vi "BMU诊断标定.vi"(8 "CAN端口":u16(ring), 9 "设备索引号":u16(ring), 10 "CAN卡类型":u32(ring)=21) -> ()   [LabVIEW 2013] (continued)
          event "保存主板参数": Value Change {
            n1903 = event-data() -> ("NewVal"=w2321:bool)  [unwired: 6 out]
            n1904 = case shown="真" w2321 {
              tunnel: w2325 -> [w2327 w2332]
              tunnel: [w2327 w2331] -> w2324
              tunnel: w2323 -> [w2326 w2330]
              tunnel: [w2326 w2329] -> w2322
              frame False {
              }
              frame True {
                n1905 = call <vilib>:"Set Busy.vi"() -> ()  [unwired: 4 in, 8 out]
                n1906 = Enqueue Element(queue=w2332, element="写配置文件", error in (no error)=w2330) -> (queue out=w2331:refnum<queue>, error out=w2329:errorcluster)  [unwired: 2 out]
              }
            }
          }
          event "继电器全开": Value Change {
            n1907 = event-data() -> ("NewVal"=w2333:bool)  [unwired: 6 out]
            n1908 = case shown="真" w2333 {
              tunnel: w2333 -> [_ w2336]
              frame False {
              }
              frame True {
                n1909 = stacked-sequence {
                  tunnel: w2336 -> [_ w2346 _]
                  frame #0 {
                    w2337 = FALSE ("清BUFF")
                    n1910 = local write "正级继电器"(w2337) -> ()
                    n1911 = local write "负级继电器"(w2337) -> ()
                    n1912 = local write "充电继电器"(w2337) -> ()
                    n1913 = local write "加热继电器"(w2337) -> ()
                    n1914 = local write "风机继电器"(w2337) -> ()
                    n1915 = local write "预充电继电器"(w2337) -> ()
                    n1916 = local write "继电器超时处理"(FALSE ("继电器超时处理")) -> ()
                    n1917 = local write "主从选择"(enum32{"主板", "从板"}."主板" ("主从选择")) -> ()
                    n1918 = local write "清BUFF"(FALSE ("清BUFF")) -> ()
                  }
                  frame #1 {
                    n1919 = case shown="真" w2346 {
                      selector: w2346 -> [_ w2361]
                      frame False {
                      }
                      frame True {
                        w2357 = 256.0 ("y")
                        w2348 = u32 1 ("命令序号")
                        w2347 = u8 192 ("命令")
                        n1920 = local read "动作保持时间"() -> (w2358:dbl)
                        n1921 = Quotient & Remainder(x=w2358, y=w2357) -> (x-y*floor(x/y)=w2350:dbl, floor(x/y)=w2354:dbl)
                        n1922 = Quotient & Remainder(x=w2354, y=w2357) -> (x-y*floor(x/y)=w2351:dbl, floor(x/y)=w2355:dbl)
                        n1923 = Quotient & Remainder(x=w2355, y=w2357) -> (x-y*floor(x/y)=w2352:dbl, floor(x/y)=w2356:dbl)
                        n1924 = local read "设备索引号"() -> (w2365:u16)
                        n1925 = local read "CAN卡类型"() -> (w2366:u32)
                        n1926 = local read "CAN端口"() -> (w2364:u16)
                        n1927 = Boolean To (0,1)(Boolean=w2361) -> (0, 1=w2359:i16)
                        n1928 = Quotient & Remainder(x=w2356, y=w2357) -> (x-y*floor(x/y)=w2353:dbl)  [unwired: 1 out]
                        n1929 = Build Array(i16 170 ("元素"), w2359, w2353, w2352, w2351, w2350, 0.0 ("元素")) -> (w2362:dbl[])
                        n1930 = call "多帧发送机制(EV05).vi"("can卡类型"=w2366, "设备索引号"=w2365, "CAN端口"=w2364, "命令"=w2347, "板号"=u8 0, "命令序号"=w2348, "输入数据"=w2362) -> ()  [unwired: 1 in, 12 out]
                        n1931 = local write "命令序号"(w2348) -> ()
                        n1932 = local write "命令"(w2347) -> ()
                      }
                    }
                    n1933 = local write "控制1"(TRUE ("控制1")) -> ()
                    n1934 = local write "写?"(FALSE ("写?")) -> ()
                    n1935 = local write "消除"(TRUE ("消除")) -> ()
                    n1936 = global write "EV05全局变量1.vi" "流控帧 2"(TRUE ("流控帧 2")) -> ()
                    n1937 = global write "EV05全局变量1.vi" "流控帧"(FALSE ("流控帧")) -> ()
                  }
                  frame #2 {
                    n1938 = flat-sequence {
                      tunnel: [w2368] -> w2367
                      tunnel: w2367 -> [w2375]
                      frame #0 {
                        n1939 = while {
                          tunnel: [w2369] -> w2368
                          i -> [w2373]
                          stop <- w2370 stop-if-true
                          n1940 = local read "继电器超时处理"() -> (w2369:bool)
                          n1941 = Greater Or Equal?(x=w2373, y=20) -> (x >= y?=w2371:bool)
                          n1942 = Wait Until Next ms Multiple(millisecond multiple=u32 100 ("毫秒倍数")) -> ()  [unwired: 1 out]
                          n1943 = Or(x=w2369, y=w2371) -> (x .or. y?=w2370:bool)
                        }
                      }
                      frame #1 {
                        n1944 = case shown="真" w2375 {
                          frame False {
                            n1945 = One Button Dialog(message="继电器处理超时" ("消息"), button name ("OK")="是" ("按钮名称（“确定”）")) -> ()  [unwired: 1 out]
                          }
                          frame True {
                            w2378 = TRUE ("清BUFF")
                            n1946 = local write "正级继电器"(w2378) -> ()
                            n1947 = local write "负级继电器"(w2378) -> ()
                            n1948 = local write "充电继电器"(w2378) -> ()
                            n1949 = local write "加热继电器"(w2378) -> ()
                            n1950 = local write "风机继电器"(w2378) -> ()
                            n1951 = local write "预充电继电器"(w2378) -> ()
                          }
                        }
                      }
                    }
                  }
                }
              }
            }
          }
          event "继电器全关": Value Change {
            n1952 = event-data() -> ("NewVal"=w2379:bool)  [unwired: 6 out]
            n1953 = case shown="真" w2379 {
              tunnel: w2379 -> [_ w2382]
              frame False {
              }
              frame True {
                n1954 = stacked-sequence {
                  tunnel: w2382 -> [_ w2392 _]
                  frame #0 {
                    w2383 = TRUE ("清BUFF")
                    n1955 = local write "正级继电器"(w2383) -> ()
                    n1956 = local write "负级继电器"(w2383) -> ()
                    n1957 = local write "充电继电器"(w2383) -> ()
                    n1958 = local write "加热继电器"(w2383) -> ()
                    n1959 = local write "风机继电器"(w2383) -> ()
                    n1960 = local write "预充电继电器"(w2383) -> ()
                    n1961 = local write "继电器超时处理"(FALSE ("继电器超时处理")) -> ()
                    n1962 = local write "主从选择"(enum32{"主板", "从板"}."主板" ("主从选择")) -> ()
                    n1963 = global write "EV05全局变量1.vi" "流控帧"(FALSE ("流控帧")) -> ()
                    n1964 = local write "清BUFF"(FALSE ("清BUFF")) -> ()
                  }
                  frame #1 {
                    n1965 = case shown="真" w2392 {
                      selector: w2392 -> [_ w2407]
                      frame False {
                      }
                      frame True {
                        w2403 = 256.0 ("y")
                        w2394 = u32 1 ("命令序号")
                        w2393 = u8 192 ("命令")
                        n1966 = local read "动作保持时间"() -> (w2404:dbl)
                        n1967 = Quotient & Remainder(x=w2404, y=w2403) -> (x-y*floor(x/y)=w2396:dbl, floor(x/y)=w2400:dbl)
                        n1968 = Quotient & Remainder(x=w2400, y=w2403) -> (x-y*floor(x/y)=w2397:dbl, floor(x/y)=w2401:dbl)
                        n1969 = Quotient & Remainder(x=w2401, y=w2403) -> (x-y*floor(x/y)=w2398:dbl, floor(x/y)=w2402:dbl)
                        n1970 = local read "设备索引号"() -> (w2411:u16)
                        n1971 = local read "CAN卡类型"() -> (w2412:u32)
                        n1972 = local read "CAN端口"() -> (w2410:u16)
                        n1973 = Boolean To (0,1)(Boolean=w2407) -> (0, 1=w2405:i16)
                        n1974 = Quotient & Remainder(x=w2402, y=w2403) -> (x-y*floor(x/y)=w2399:dbl)  [unwired: 1 out]
                        n1975 = Build Array(i16 85 ("元素"), w2405, w2399, w2398, w2397, w2396, 0.0 ("元素")) -> (w2408:dbl[])
                        n1976 = call "多帧发送机制(EV05).vi"("can卡类型"=w2412, "设备索引号"=w2411, "CAN端口"=w2410, "命令"=w2393, "板号"=u8 0, "命令序号"=w2394, "输入数据"=w2408) -> ()  [unwired: 1 in, 12 out]
                        n1977 = local write "命令序号"(w2394) -> ()
                        n1978 = local write "命令"(w2393) -> ()
                      }
                    }
                    n1979 = local write "控制1"(TRUE ("控制1")) -> ()
                    n1980 = local write "写?"(FALSE ("写?")) -> ()
                    n1981 = local write "消除"(TRUE ("消除")) -> ()
                    n1982 = global write "EV05全局变量1.vi" "流控帧 2"(TRUE ("流控帧 2")) -> ()
                  }
                  frame #2 {
                    n1983 = flat-sequence {
                      tunnel: [w2414] -> w2413
                      tunnel: w2413 -> [w2421]
                      frame #0 {
                        n1984 = while {
                          tunnel: [w2415] -> w2414
                          i -> [w2419]
                          stop <- w2416 stop-if-true
                          n1985 = local read "继电器超时处理"() -> (w2415:bool)
                          n1986 = Greater Or Equal?(x=w2419, y=20) -> (x >= y?=w2417:bool)
                          n1987 = Wait Until Next ms Multiple(millisecond multiple=u32 100 ("毫秒倍数")) -> ()  [unwired: 1 out]
                          n1988 = Or(x=w2415, y=w2417) -> (x .or. y?=w2416:bool)
                        }
                      }
                      frame #1 {
                        n1989 = case shown="真" w2421 {
                          frame False {
                            n1990 = One Button Dialog(message="继电器处理超时" ("消息"), button name ("OK")="是" ("按钮名称（“确定”）")) -> ()  [unwired: 1 out]
                          }
                          frame True {
                            w2424 = FALSE ("清BUFF")
                            n1991 = local write "正级继电器"(w2424) -> ()
                            n1992 = local write "负级继电器"(w2424) -> ()
                            n1993 = local write "充电继电器"(w2424) -> ()
                            n1994 = local write "加热继电器"(w2424) -> ()
                            n1995 = local write "风机继电器"(w2424) -> ()
                            n1996 = local write "预充电继电器"(w2424) -> ()
                          }
                        }
                      }
                    }
                  }
                }
              }
            }
          }
          event "控制按键全为开": Value Change {
            n1997 = event-data() -> ("NewVal"=w2425:bool)  [unwired: 6 out]
            n1998 = case shown="真" w2425 {
              frame False {
              }
              frame True {
                w2426 = TRUE ("正级继电器")
                n1999 = local write "加热继电器(从)"(w2426) -> ()
                n2000 = local write "风机继电器(从)"(w2426) -> ()
                n2001 = local write "DO1 2"(w2426) -> ()
                n2002 = local write "DO1"(w2426) -> ()
                n2003 = local write "DO2"(w2426) -> ()
                n2004 = local write "正级继电器"(w2426) -> ()
                n2005 = local write "负级继电器"(w2426) -> ()
                n2006 = local write "加热继电器"(w2426) -> ()
                n2007 = local write "预充电继电器"(w2426) -> ()
                n2008 = local write "充电继电器"(w2426) -> ()
                n2009 = local write "风机继电器"(w2426) -> ()
              }
            }
          }
          event "控制按键全为关": Value Change {
            n2010 = event-data() -> ("NewVal"=w2427:bool)  [unwired: 6 out]
            n2011 = case shown="真" w2427 {
              frame False {
              }
              frame True {
                w2428 = FALSE ("正级继电器")
                n2012 = local write "加热继电器(从)"(w2428) -> ()
                n2013 = local write "风机继电器(从)"(w2428) -> ()
                n2014 = local write "DO1 2"(w2428) -> ()
                n2015 = local write "DO1"(w2428) -> ()
                n2016 = local write "DO2"(w2428) -> ()
                n2017 = local write "正级继电器"(w2428) -> ()
                n2018 = local write "负级继电器"(w2428) -> ()
                n2019 = local write "加热继电器"(w2428) -> ()
                n2020 = local write "预充电继电器"(w2428) -> ()
                n2021 = local write "充电继电器"(w2428) -> ()
                n2022 = local write "风机继电器"(w2428) -> ()
              }
            }
          }
          event "正级继电器": Value Change {
            n2023 = event-data() -> ("NewVal"=w2429:bool)  [unwired: 6 out]
            n2024 = stacked-sequence {
              tunnel: w2429 -> [_ w2442 _]
              frame #0 {
                w2432 = FALSE ("清BUFF")
                n2025 = local write "继电器超时处理"(FALSE ("继电器超时处理")) -> ()
                n2026 = local write "主从选择"(enum32{"主板", "从板"}."主板" ("主从选择")) -> ()
                n2027 = local write "正级继电器 12"(w2432) -> ()
                n2028 = local write "清BUFF"(w2432) -> ()
              }
              frame #1 {
                n2029 = case shown="假" w2442 {
                  selector: w2442 -> [w2457 w2477]
                  tunnel: [w2456 w2476] -> w2441
                  tunnel: [w2444 w2464] -> w2436
                  frame False {
                    w2452 = 256.0 ("y")
                    w2444 = u32 1 ("命令序号")
                    w2456 = u8 192 ("命令")
                    n2030 = local read "动作保持时间"() -> (w2453:dbl)
                    n2031 = Quotient & Remainder(x=w2453, y=w2452) -> (x-y*floor(x/y)=w2445:dbl, floor(x/y)=w2449:dbl)
                    n2032 = Quotient & Remainder(x=w2449, y=w2452) -> (x-y*floor(x/y)=w2446:dbl, floor(x/y)=w2450:dbl)
                    n2033 = Quotient & Remainder(x=w2450, y=w2452) -> (x-y*floor(x/y)=w2447:dbl, floor(x/y)=w2451:dbl)
                    n2034 = local read "设备索引号"() -> (w2461:u16)
                    n2035 = local read "CAN卡类型"() -> (w2462:u32)
                    n2036 = local read "CAN端口"() -> (w2460:u16)
                    n2037 = Boolean To (0,1)(Boolean=w2457) -> (0, 1=w2454:i16)
                    n2038 = Quotient & Remainder(x=w2451, y=w2452) -> (x-y*floor(x/y)=w2448:dbl)  [unwired: 1 out]
                    n2039 = Build Array(i16 1 ("元素"), w2454, w2448, w2447, w2446, w2445, 0.0 ("元素")) -> (w2458:dbl[])
                    n2040 = call "多帧发送机制(EV05).vi"("can卡类型"=w2462, "设备索引号"=w2461, "CAN端口"=w2460, "命令"=w2456, "板号"=u8 0, "命令序号"=w2444, "输入数据"=w2458) -> ()  [unwired: 1 in, 12 out]
                  }
                  frame True {
                    w2472 = 256.0 ("y")
                    w2464 = u32 1 ("命令序号")
                    w2476 = u8 192 ("命令")
                    n2041 = local read "动作保持时间"() -> (w2473:dbl)
                    n2042 = Quotient & Remainder(x=w2473, y=w2472) -> (x-y*floor(x/y)=w2465:dbl, floor(x/y)=w2469:dbl)
                    n2043 = Quotient & Remainder(x=w2469, y=w2472) -> (x-y*floor(x/y)=w2466:dbl, floor(x/y)=w2470:dbl)
                    n2044 = Quotient & Remainder(x=w2470, y=w2472) -> (x-y*floor(x/y)=w2467:dbl, floor(x/y)=w2471:dbl)
                    n2045 = local read "设备索引号"() -> (w2481:u16)
                    n2046 = local read "CAN卡类型"() -> (w2482:u32)
                    n2047 = local read "CAN端口"() -> (w2480:u16)
                    n2048 = Boolean To (0,1)(Boolean=w2477) -> (0, 1=w2474:i16)
                    n2049 = Quotient & Remainder(x=w2471, y=w2472) -> (x-y*floor(x/y)=w2468:dbl)  [unwired: 1 out]
                    n2050 = Build Array(i16 1 ("元素"), w2474, w2468, w2467, w2466, w2465, 0.0 ("元素")) -> (w2478:dbl[])
                    n2051 = call "多帧发送机制(EV05).vi"("can卡类型"=w2482, "设备索引号"=w2481, "CAN端口"=w2480, "命令"=w2476, "板号"=u8 0, "命令序号"=w2464, "输入数据"=w2478) -> ()  [unwired: 1 in, 12 out]
                  }
                }
                n2052 = local write "命令序号"(w2436) -> ()
                n2053 = local write "命令"(w2441) -> ()
                n2054 = local write "控制1"(TRUE ("控制1")) -> ()
                n2055 = local write "写?"(FALSE ("写?")) -> ()
                n2056 = global write "EV05全局变量1.vi" "流控帧"(FALSE ("流控帧")) -> ()
                n2057 = local write "消除"(TRUE ("消除")) -> ()
                n2058 = global write "EV05全局变量1.vi" "流控帧 2"(TRUE ("流控帧 2")) -> ()
              }
              frame #2 {
                n2059 = flat-sequence {
                  tunnel: [w2484] -> w2483
                  tunnel: w2483 -> [w2491]
                  frame #0 {
                    n2060 = while {
                      tunnel: [w2485] -> w2484
                      i -> [w2489]
                      stop <- w2486 stop-if-true
                      n2061 = local read "继电器超时处理"() -> (w2485:bool)
                      n2062 = Greater Or Equal?(x=w2489, y=20) -> (x >= y?=w2487:bool)
                      n2063 = Wait Until Next ms Multiple(millisecond multiple=u32 100 ("毫秒倍数")) -> ()  [unwired: 1 out]
                      n2064 = Or(x=w2485, y=w2487) -> (x .or. y?=w2486:bool)
                    }
                  }
                  frame #1 {
                    n2065 = case shown="假" w2491 {
                      frame False {
                        n2066 = local read "正级继电器"() -> (w2493:bool)
                        n2067 = Not(x=w2493) -> (.not. x?=w2492:bool)
                        n2068 = local write "正级继电器"(w2492) -> ()
                        n2069 = One Button Dialog(message="继电器处理超时" ("消息"), button name ("OK")="是" ("按钮名称（“确定”）")) -> ()  [unwired: 1 out]
                      }
                      frame True {
                      }
                    }
                  }
                }
              }
            }
          }
          event "负级继电器": Value Change {
            n2070 = event-data() -> ("NewVal"=w2496:bool)  [unwired: 6 out]
            n2071 = stacked-sequence {
              tunnel: w2496 -> [_ w2509 _]
              frame #0 {
                w2499 = FALSE ("继电器超时处理")
                n2072 = local write "继电器超时处理"(w2499) -> ()
                n2073 = local write "正级继电器 2"(w2499) -> ()
                n2074 = local write "主从选择"(enum32{"主板", "从板"}."主板" ("主从选择")) -> ()
              }
              frame #1 {
                n2075 = case shown="假" w2509 {
                  selector: w2509 -> [w2523 w2543]
                  tunnel: [w2522 w2542] -> w2508
                  tunnel: [w2511 w2531] -> w2503
                  frame False {
                    w2519 = 256.0 ("y")
                    w2511 = u32 1 ("命令序号")
                    w2522 = u8 192 ("命令")
                    n2076 = local read "动作保持时间"() -> (w2520:dbl)
                    n2077 = Quotient & Remainder(x=w2520, y=w2519) -> (x-y*floor(x/y)=w2512:dbl, floor(x/y)=w2516:dbl)
                    n2078 = Quotient & Remainder(x=w2516, y=w2519) -> (x-y*floor(x/y)=w2513:dbl, floor(x/y)=w2517:dbl)
                    n2079 = Quotient & Remainder(x=w2517, y=w2519) -> (x-y*floor(x/y)=w2514:dbl, floor(x/y)=w2518:dbl)
                    n2080 = Quotient & Remainder(x=w2518, y=w2519) -> (x-y*floor(x/y)=w2515:dbl)  [unwired: 1 out]
                    n2081 = Boolean To (0,1)(Boolean=w2523) -> (0, 1=w2521:i16)
                    n2082 = local read "设备索引号"() -> (w2528:u16)
                    n2083 = local read "CAN卡类型"() -> (w2529:u32)
                    n2084 = local read "CAN端口"() -> (w2527:u16)
                    n2085 = Build Array(i16 2 ("元素"), w2521, w2515, w2514, w2513, w2512, 0.0 ("元素")) -> (w2525:dbl[])
                    n2086 = call "多帧发送机制(EV05).vi"("can卡类型"=w2529, "设备索引号"=w2528, "CAN端口"=w2527, "命令"=w2522, "板号"=u8 0, "命令序号"=w2511, "输入数据"=w2525) -> ()  [unwired: 1 in, 12 out]
                  }
                  frame True {
                    w2539 = 256.0 ("y")
                    w2531 = u32 1 ("命令序号")
                    w2542 = u8 192 ("命令")
                    n2087 = local read "动作保持时间"() -> (w2540:dbl)
                    n2088 = Quotient & Remainder(x=w2540, y=w2539) -> (x-y*floor(x/y)=w2532:dbl, floor(x/y)=w2536:dbl)
                    n2089 = Quotient & Remainder(x=w2536, y=w2539) -> (x-y*floor(x/y)=w2533:dbl, floor(x/y)=w2537:dbl)
                    n2090 = Quotient & Remainder(x=w2537, y=w2539) -> (x-y*floor(x/y)=w2534:dbl, floor(x/y)=w2538:dbl)
                    n2091 = Quotient & Remainder(x=w2538, y=w2539) -> (x-y*floor(x/y)=w2535:dbl)  [unwired: 1 out]
                    n2092 = Boolean To (0,1)(Boolean=w2543) -> (0, 1=w2541:i16)
                    n2093 = local read "设备索引号"() -> (w2548:u16)
                    n2094 = local read "CAN卡类型"() -> (w2549:u32)
                    n2095 = local read "CAN端口"() -> (w2547:u16)
                    n2096 = Build Array(i16 2 ("元素"), w2541, w2535, w2534, w2533, w2532, 0.0 ("元素")) -> (w2545:dbl[])
                    n2097 = call "多帧发送机制(EV05).vi"("can卡类型"=w2549, "设备索引号"=w2548, "CAN端口"=w2547, "命令"=w2542, "板号"=u8 0, "命令序号"=w2531, "输入数据"=w2545) -> ()  [unwired: 1 in, 12 out]
                  }
                }
                n2098 = local write "命令"(w2508) -> ()
                n2099 = local write "命令序号"(w2503) -> ()
                n2100 = local write "清BUFF"(FALSE ("清BUFF")) -> ()
                n2101 = global write "EV05全局变量1.vi" "流控帧"(FALSE ("流控帧")) -> ()
                n2102 = local write "控制1"(TRUE ("控制1")) -> ()
                n2103 = global write "EV05全局变量1.vi" "流控帧 2"(TRUE ("流控帧 2")) -> ()
                n2104 = local write "写?"(FALSE ("写?")) -> ()
                n2105 = local write "消除"(TRUE ("消除")) -> ()
              }
              frame #2 {
                n2106 = flat-sequence {
                  tunnel: [w2551] -> w2550
                  tunnel: w2550 -> [w2558]
                  frame #0 {
                    n2107 = while {
                      tunnel: [w2552] -> w2551
                      i -> [w2556]
                      stop <- w2553 stop-if-true
                      n2108 = local read "继电器超时处理"() -> (w2552:bool)
                      n2109 = Greater Or Equal?(x=w2556, y=20) -> (x >= y?=w2554:bool)
                      n2110 = Wait Until Next ms Multiple(millisecond multiple=u32 100 ("毫秒倍数")) -> ()  [unwired: 1 out]
                      n2111 = Or(x=w2552, y=w2554) -> (x .or. y?=w2553:bool)
                    }
                  }
                  frame #1 {
                    n2112 = case shown="假" w2558 {
                      frame False {
                        n2113 = local read "负级继电器"() -> (w2559:bool)
                        n2114 = Not(x=w2559) -> (.not. x?=w2560:bool)
                        n2115 = local write "负级继电器"(w2560) -> ()
                        n2116 = One Button Dialog(message="继电器处理超时" ("消息"), button name ("OK")="是" ("按钮名称（“确定”）")) -> ()  [unwired: 1 out]
                      }
                      frame True {
                      }
                    }
                  }
                }
              }
            }
          }
          event "预充电继电器": Value Change {
            n2117 = event-data() -> ("NewVal"=w2563:bool)  [unwired: 6 out]
            n2118 = stacked-sequence {
              tunnel: w2563 -> [_ w2576 _]
              frame #0 {
                w2567 = FALSE ("继电器超时处理")
                n2119 = local write "继电器超时处理"(w2567) -> ()
                n2120 = local write "正级继电器 3"(w2567) -> ()
                n2121 = global write "EV05全局变量1.vi" "流控帧"(FALSE ("流控帧")) -> ()
                n2122 = local write "主从选择"(enum32{"主板", "从板"}."主板" ("主从选择")) -> ()
              }
              frame #1 {
                n2123 = case shown="假" w2576 {
                  selector: w2576 -> [w2590 w2610]
                  tunnel: [w2589 w2609] -> w2575
                  tunnel: [w2578 w2598] -> w2570
                  frame False {
                    w2586 = 256.0 ("y")
                    w2578 = u32 1 ("命令序号")
                    w2589 = u8 192 ("命令")
                    n2124 = local read "动作保持时间"() -> (w2587:dbl)
                    n2125 = Quotient & Remainder(x=w2587, y=w2586) -> (x-y*floor(x/y)=w2579:dbl, floor(x/y)=w2583:dbl)
                    n2126 = Quotient & Remainder(x=w2583, y=w2586) -> (x-y*floor(x/y)=w2580:dbl, floor(x/y)=w2584:dbl)
                    n2127 = Quotient & Remainder(x=w2584, y=w2586) -> (x-y*floor(x/y)=w2581:dbl, floor(x/y)=w2585:dbl)
                    n2128 = Quotient & Remainder(x=w2585, y=w2586) -> (x-y*floor(x/y)=w2582:dbl)  [unwired: 1 out]
                    n2129 = Boolean To (0,1)(Boolean=w2590) -> (0, 1=w2588:i16)
                    n2130 = local read "设备索引号"() -> (w2595:u16)
                    n2131 = local read "CAN卡类型"() -> (w2596:u32)
                    n2132 = local read "CAN端口"() -> (w2594:u16)
                    n2133 = Build Array(i16 3 ("元素"), w2588, w2582, w2581, w2580, w2579, 0.0 ("元素")) -> (w2592:dbl[])
                    n2134 = call "多帧发送机制(EV05).vi"("can卡类型"=w2596, "设备索引号"=w2595, "CAN端口"=w2594, "命令"=w2589, "板号"=u8 0, "命令序号"=w2578, "输入数据"=w2592) -> ()  [unwired: 1 in, 12 out]
                  }
                  frame True {
                    w2606 = 256.0 ("y")
                    w2598 = u32 1 ("命令序号")
                    w2609 = u8 192 ("命令")
                    n2135 = local read "动作保持时间"() -> (w2607:dbl)
                    n2136 = Quotient & Remainder(x=w2607, y=w2606) -> (x-y*floor(x/y)=w2599:dbl, floor(x/y)=w2603:dbl)
                    n2137 = Quotient & Remainder(x=w2603, y=w2606) -> (x-y*floor(x/y)=w2600:dbl, floor(x/y)=w2604:dbl)
                    n2138 = Quotient & Remainder(x=w2604, y=w2606) -> (x-y*floor(x/y)=w2601:dbl, floor(x/y)=w2605:dbl)
                    n2139 = Quotient & Remainder(x=w2605, y=w2606) -> (x-y*floor(x/y)=w2602:dbl)  [unwired: 1 out]
                    n2140 = Boolean To (0,1)(Boolean=w2610) -> (0, 1=w2608:i16)
                    n2141 = local read "设备索引号"() -> (w2615:u16)
                    n2142 = local read "CAN卡类型"() -> (w2616:u32)
                    n2143 = local read "CAN端口"() -> (w2614:u16)
                    n2144 = Build Array(i16 3 ("元素"), w2608, w2602, w2601, w2600, w2599, 0.0 ("元素")) -> (w2612:dbl[])
                    n2145 = call "多帧发送机制(EV05).vi"("can卡类型"=w2616, "设备索引号"=w2615, "CAN端口"=w2614, "命令"=w2609, "板号"=u8 0, "命令序号"=w2598, "输入数据"=w2612) -> ()  [unwired: 1 in, 12 out]
                  }
                }
                n2146 = local write "命令序号"(w2570) -> ()
                n2147 = local write "清BUFF"(FALSE ("清BUFF")) -> ()
                n2148 = local write "控制1"(TRUE ("控制1")) -> ()
                n2149 = global write "EV05全局变量1.vi" "流控帧 2"(TRUE ("流控帧 2")) -> ()
                n2150 = local write "消除"(TRUE ("消除")) -> ()
                n2151 = local write "命令"(w2575) -> ()
                n2152 = local write "写?"(FALSE ("写?")) -> ()
              }
              frame #2 {
                n2153 = flat-sequence {
                  tunnel: [w2618] -> w2617
                  tunnel: w2617 -> [w2625]
                  frame #0 {
                    n2154 = while {
                      tunnel: [w2619] -> w2618
                      i -> [w2623]
                      stop <- w2620 stop-if-true
                      n2155 = local read "继电器超时处理"() -> (w2619:bool)
                      n2156 = Greater Or Equal?(x=w2623, y=20) -> (x >= y?=w2621:bool)
                      n2157 = Wait Until Next ms Multiple(millisecond multiple=u32 100 ("毫秒倍数")) -> ()  [unwired: 1 out]
                      n2158 = Or(x=w2619, y=w2621) -> (x .or. y?=w2620:bool)
                    }
                  }
                  frame #1 {
                    n2159 = case shown="假" w2625 {
                      frame False {
                        n2160 = local read "预充电继电器"() -> (w2626:bool)
                        n2161 = Not(x=w2626) -> (.not. x?=w2627:bool)
                        n2162 = local write "预充电继电器"(w2627) -> ()
                        n2163 = One Button Dialog(message="继电器处理超时" ("消息"), button name ("OK")="是" ("按钮名称（“确定”）")) -> ()  [unwired: 1 out]
                      }
                      frame True {
                      }
                    }
                  }
                }
              }
            }
          }
          event "加热继电器": Value Change {
            n2164 = event-data() -> ("NewVal"=w2630:bool)  [unwired: 6 out]
            n2165 = stacked-sequence {
              tunnel: w2630 -> [_ w2643 _]
              frame #0 {
                w2634 = FALSE ("继电器超时处理")
                n2166 = local write "继电器超时处理"(w2634) -> ()
                n2167 = local write "正级继电器 5"(w2634) -> ()
                n2168 = global write "EV05全局变量1.vi" "流控帧"(FALSE ("流控帧")) -> ()
                n2169 = local write "主从选择"(enum32{"主板", "从板"}."主板" ("主从选择")) -> ()
              }
              frame #1 {
                n2170 = case shown="假" w2643 {
                  selector: w2643 -> [w2657 w2677]
                  tunnel: [w2656 w2676] -> w2642
                  tunnel: [w2645 w2665] -> w2637
                  frame False {
                    w2653 = 256.0 ("y")
                    w2645 = u32 1 ("命令序号")
                    w2656 = u8 192 ("命令")
                    n2171 = local read "动作保持时间"() -> (w2654:dbl)
                    n2172 = Quotient & Remainder(x=w2654, y=w2653) -> (x-y*floor(x/y)=w2646:dbl, floor(x/y)=w2650:dbl)
                    n2173 = Quotient & Remainder(x=w2650, y=w2653) -> (x-y*floor(x/y)=w2647:dbl, floor(x/y)=w2651:dbl)
                    n2174 = Quotient & Remainder(x=w2651, y=w2653) -> (x-y*floor(x/y)=w2648:dbl, floor(x/y)=w2652:dbl)
                    n2175 = Quotient & Remainder(x=w2652, y=w2653) -> (x-y*floor(x/y)=w2649:dbl)  [unwired: 1 out]
                    n2176 = Boolean To (0,1)(Boolean=w2657) -> (0, 1=w2655:i16)
                    n2177 = local read "设备索引号"() -> (w2662:u16)
                    n2178 = local read "CAN卡类型"() -> (w2663:u32)
                    n2179 = local read "CAN端口"() -> (w2661:u16)
                    n2180 = Build Array(i16 4 ("元素"), w2655, w2649, w2648, w2647, w2646, 0.0 ("元素")) -> (w2659:dbl[])
                    n2181 = call "多帧发送机制(EV05).vi"("can卡类型"=w2663, "设备索引号"=w2662, "CAN端口"=w2661, "命令"=w2656, "板号"=u8 0, "命令序号"=w2645, "输入数据"=w2659) -> ()  [unwired: 1 in, 12 out]
                  }
                  frame True {
                    w2673 = 256.0 ("y")
                    w2665 = u32 1 ("命令序号")
                    w2676 = u8 192 ("命令")
                    n2182 = local read "动作保持时间"() -> (w2674:dbl)
                    n2183 = Quotient & Remainder(x=w2674, y=w2673) -> (x-y*floor(x/y)=w2666:dbl, floor(x/y)=w2670:dbl)
                    n2184 = Quotient & Remainder(x=w2670, y=w2673) -> (x-y*floor(x/y)=w2667:dbl, floor(x/y)=w2671:dbl)
                    n2185 = Quotient & Remainder(x=w2671, y=w2673) -> (x-y*floor(x/y)=w2668:dbl, floor(x/y)=w2672:dbl)
                    n2186 = Quotient & Remainder(x=w2672, y=w2673) -> (x-y*floor(x/y)=w2669:dbl)  [unwired: 1 out]
                    n2187 = Boolean To (0,1)(Boolean=w2677) -> (0, 1=w2675:i16)
                    n2188 = local read "设备索引号"() -> (w2682:u16)
                    n2189 = local read "CAN卡类型"() -> (w2683:u32)
                    n2190 = local read "CAN端口"() -> (w2681:u16)
                    n2191 = Build Array(i16 4 ("元素"), w2675, w2669, w2668, w2667, w2666, 0.0 ("元素")) -> (w2679:dbl[])
                    n2192 = call "多帧发送机制(EV05).vi"("can卡类型"=w2683, "设备索引号"=w2682, "CAN端口"=w2681, "命令"=w2676, "板号"=u8 0, "命令序号"=w2665, "输入数据"=w2679) -> ()  [unwired: 1 in, 12 out]
                  }
                }
                n2193 = local write "命令序号"(w2637) -> ()
                n2194 = local write "清BUFF"(FALSE ("清BUFF")) -> ()
                n2195 = local write "命令"(w2642) -> ()
                n2196 = local write "控制1"(TRUE ("控制1")) -> ()
                n2197 = local write "写?"(FALSE ("写?")) -> ()
                n2198 = global write "EV05全局变量1.vi" "流控帧 2"(TRUE ("流控帧 2")) -> ()
                n2199 = local write "消除"(TRUE ("消除")) -> ()
              }
              frame #2 {
                n2200 = flat-sequence {
                  tunnel: [w2685] -> w2684
                  tunnel: w2684 -> [w2692]
                  frame #0 {
                    n2201 = while {
                      tunnel: [w2686] -> w2685
                      i -> [w2690]
                      stop <- w2687 stop-if-true
                      n2202 = local read "继电器超时处理"() -> (w2686:bool)
                      n2203 = Greater Or Equal?(x=w2690, y=20) -> (x >= y?=w2688:bool)
                      n2204 = Wait Until Next ms Multiple(millisecond multiple=u32 100 ("毫秒倍数")) -> ()  [unwired: 1 out]
                      n2205 = Or(x=w2686, y=w2688) -> (x .or. y?=w2687:bool)
                    }
                  }
                  frame #1 {
                    n2206 = case shown="假" w2692 {
                      frame False {
                        n2207 = local read "加热继电器"() -> (w2693:bool)
                        n2208 = Not(x=w2693) -> (.not. x?=w2694:bool)
                        n2209 = local write "加热继电器"(w2694) -> ()
                        n2210 = One Button Dialog(message="继电器处理超时" ("消息"), button name ("OK")="是" ("按钮名称（“确定”）")) -> ()  [unwired: 1 out]
                      }
                      frame True {
                      }
                    }
                  }
                }
              }
            }
          }
          event "充电继电器": Value Change {
            n2211 = event-data() -> ("NewVal"=w2697:bool)  [unwired: 6 out]
            n2212 = stacked-sequence {
              tunnel: w2697 -> [_ w2710 _]
              frame #0 {
                w2701 = FALSE ("继电器超时处理")
                n2213 = local write "主从选择"(enum32{"主板", "从板"}."主板" ("主从选择")) -> ()
                n2214 = global write "EV05全局变量1.vi" "流控帧"(FALSE ("流控帧")) -> ()
                n2215 = local write "继电器超时处理"(w2701) -> ()
                n2216 = local write "正级继电器 4"(w2701) -> ()
              }
              frame #1 {
                n2217 = case shown="假" w2710 {
                  selector: w2710 -> [w2724 w2744]
                  tunnel: [w2723 w2743] -> w2709
                  tunnel: [w2712 w2732] -> w2704
                  frame False {
                    w2720 = 256.0 ("y")
                    w2712 = u32 1 ("命令序号")
                    w2723 = u8 192 ("命令")
                    n2218 = local read "动作保持时间"() -> (w2721:dbl)
                    n2219 = Quotient & Remainder(x=w2721, y=w2720) -> (x-y*floor(x/y)=w2713:dbl, floor(x/y)=w2717:dbl)
                    n2220 = Quotient & Remainder(x=w2717, y=w2720) -> (x-y*floor(x/y)=w2714:dbl, floor(x/y)=w2718:dbl)
                    n2221 = Quotient & Remainder(x=w2718, y=w2720) -> (x-y*floor(x/y)=w2715:dbl, floor(x/y)=w2719:dbl)
                    n2222 = Quotient & Remainder(x=w2719, y=w2720) -> (x-y*floor(x/y)=w2716:dbl)  [unwired: 1 out]
                    n2223 = Boolean To (0,1)(Boolean=w2724) -> (0, 1=w2722:i16)
                    n2224 = local read "设备索引号"() -> (w2729:u16)
                    n2225 = local read "CAN卡类型"() -> (w2730:u32)
                    n2226 = local read "CAN端口"() -> (w2728:u16)
                    n2227 = Build Array(i16 5 ("元素"), w2722, w2716, w2715, w2714, w2713, 0.0 ("元素")) -> (w2726:dbl[])
                    n2228 = call "多帧发送机制(EV05).vi"("can卡类型"=w2730, "设备索引号"=w2729, "CAN端口"=w2728, "命令"=w2723, "板号"=u8 0, "命令序号"=w2712, "输入数据"=w2726) -> ()  [unwired: 1 in, 12 out]
                  }
                  frame True {
                    w2740 = 256.0 ("y")
                    w2732 = u32 1 ("命令序号")
                    w2743 = u8 192 ("命令")
                    n2229 = local read "动作保持时间"() -> (w2741:dbl)
                    n2230 = Quotient & Remainder(x=w2741, y=w2740) -> (x-y*floor(x/y)=w2733:dbl, floor(x/y)=w2737:dbl)
                    n2231 = Quotient & Remainder(x=w2737, y=w2740) -> (x-y*floor(x/y)=w2734:dbl, floor(x/y)=w2738:dbl)
                    n2232 = Quotient & Remainder(x=w2738, y=w2740) -> (x-y*floor(x/y)=w2735:dbl, floor(x/y)=w2739:dbl)
                    n2233 = Quotient & Remainder(x=w2739, y=w2740) -> (x-y*floor(x/y)=w2736:dbl)  [unwired: 1 out]
                    n2234 = Boolean To (0,1)(Boolean=w2744) -> (0, 1=w2742:i16)
                    n2235 = local read "设备索引号"() -> (w2749:u16)
                    n2236 = local read "CAN卡类型"() -> (w2750:u32)
                    n2237 = local read "CAN端口"() -> (w2748:u16)
                    n2238 = Build Array(i16 5 ("元素"), w2742, w2736, w2735, w2734, w2733, 0.0 ("元素")) -> (w2746:dbl[])
                    n2239 = call "多帧发送机制(EV05).vi"("can卡类型"=w2750, "设备索引号"=w2749, "CAN端口"=w2748, "命令"=w2743, "板号"=u8 0, "命令序号"=w2732, "输入数据"=w2746) -> ()  [unwired: 1 in, 12 out]
                  }
                }
                n2240 = local write "命令序号"(w2704) -> ()
                n2241 = local write "命令"(w2709) -> ()
                n2242 = local write "清BUFF"(FALSE ("清BUFF")) -> ()
                n2243 = local write "控制1"(TRUE ("控制1")) -> ()
                n2244 = global write "EV05全局变量1.vi" "流控帧 2"(TRUE ("流控帧 2")) -> ()
                n2245 = local write "写?"(FALSE ("写?")) -> ()
                n2246 = local write "消除"(TRUE ("消除")) -> ()
              }
              frame #2 {
                n2247 = flat-sequence {
                  tunnel: [w2752] -> w2751
                  tunnel: w2751 -> [w2759]
                  frame #0 {
                    n2248 = while {
                      tunnel: [w2753] -> w2752
                      i -> [w2757]
                      stop <- w2754 stop-if-true
                      n2249 = local read "继电器超时处理"() -> (w2753:bool)
                      n2250 = Greater Or Equal?(x=w2757, y=20) -> (x >= y?=w2755:bool)
                      n2251 = Wait Until Next ms Multiple(millisecond multiple=u32 100 ("毫秒倍数")) -> ()  [unwired: 1 out]
                      n2252 = Or(x=w2753, y=w2755) -> (x .or. y?=w2754:bool)
                    }
                  }
                  frame #1 {
                    n2253 = case shown="假" w2759 {
                      frame False {
                        n2254 = local read "充电继电器"() -> (w2760:bool)
                        n2255 = Not(x=w2760) -> (.not. x?=w2761:bool)
                        n2256 = local write "充电继电器"(w2761) -> ()
                        n2257 = One Button Dialog(message="继电器处理超时" ("消息"), button name ("OK")="是" ("按钮名称（“确定”）")) -> ()  [unwired: 1 out]
                      }
                      frame True {
                      }
                    }
                  }
                }
              }
            }
          }
          event "风机继电器": Value Change {
            n2258 = event-data() -> ("NewVal"=w2764:bool)  [unwired: 6 out]
            n2259 = stacked-sequence {
              tunnel: w2764 -> [_ w2777 _]
              frame #0 {
                w2768 = FALSE ("继电器超时处理")
                n2260 = local write "继电器超时处理"(w2768) -> ()
                n2261 = local write "正级继电器 6"(w2768) -> ()
                n2262 = global write "EV05全局变量1.vi" "流控帧"(FALSE ("流控帧")) -> ()
                n2263 = local write "主从选择"(enum32{"主板", "从板"}."主板" ("主从选择")) -> ()
              }
              frame #1 {
                n2264 = case shown="真" w2777 {
                  selector: w2777 -> [w2791 w2811]
                  tunnel: [w2790 w2810] -> w2776
                  tunnel: [w2779 w2799] -> w2771
                  frame True {
                    w2787 = 256.0 ("y")
                    w2779 = u32 1 ("命令序号")
                    w2790 = u8 192 ("命令")
                    n2265 = local read "动作保持时间"() -> (w2788:dbl)
                    n2266 = Quotient & Remainder(x=w2788, y=w2787) -> (x-y*floor(x/y)=w2780:dbl, floor(x/y)=w2784:dbl)
                    n2267 = Quotient & Remainder(x=w2784, y=w2787) -> (x-y*floor(x/y)=w2781:dbl, floor(x/y)=w2785:dbl)
                    n2268 = Quotient & Remainder(x=w2785, y=w2787) -> (x-y*floor(x/y)=w2782:dbl, floor(x/y)=w2786:dbl)
                    n2269 = Boolean To (0,1)(Boolean=w2791) -> (0, 1=w2789:i16)
                    n2270 = local read "设备索引号"() -> (w2796:u16)
                    n2271 = local read "CAN卡类型"() -> (w2797:u32)
                    n2272 = Quotient & Remainder(x=w2786, y=w2787) -> (x-y*floor(x/y)=w2783:dbl)  [unwired: 1 out]
                    n2273 = local read "CAN端口"() -> (w2795:u16)
                    n2274 = Build Array(i16 6 ("元素"), w2789, w2783, w2782, w2781, w2780, 0.0 ("元素")) -> (w2793:dbl[])
                    n2275 = call "多帧发送机制(EV05).vi"("can卡类型"=w2797, "设备索引号"=w2796, "CAN端口"=w2795, "命令"=w2790, "板号"=u8 0, "命令序号"=w2779, "输入数据"=w2793) -> ()  [unwired: 1 in, 12 out]
                  }
                  frame False {
                    w2807 = 256.0 ("y")
                    w2799 = u32 1 ("命令序号")
                    w2810 = u8 192 ("命令")
                    n2276 = local read "动作保持时间"() -> (w2808:dbl)
                    n2277 = Quotient & Remainder(x=w2808, y=w2807) -> (x-y*floor(x/y)=w2800:dbl, floor(x/y)=w2804:dbl)
                    n2278 = Quotient & Remainder(x=w2804, y=w2807) -> (x-y*floor(x/y)=w2801:dbl, floor(x/y)=w2805:dbl)
                    n2279 = Quotient & Remainder(x=w2805, y=w2807) -> (x-y*floor(x/y)=w2802:dbl, floor(x/y)=w2806:dbl)
                    n2280 = Boolean To (0,1)(Boolean=w2811) -> (0, 1=w2809:i16)
                    n2281 = local read "设备索引号"() -> (w2816:u16)
                    n2282 = local read "CAN卡类型"() -> (w2817:u32)
                    n2283 = Quotient & Remainder(x=w2806, y=w2807) -> (x-y*floor(x/y)=w2803:dbl)  [unwired: 1 out]
                    n2284 = local read "CAN端口"() -> (w2815:u16)
                    n2285 = Build Array(i16 6 ("元素"), w2809, w2803, w2802, w2801, w2800, 0.0 ("元素")) -> (w2813:dbl[])
                    n2286 = call "多帧发送机制(EV05).vi"("can卡类型"=w2817, "设备索引号"=w2816, "CAN端口"=w2815, "命令"=w2810, "板号"=u8 0, "命令序号"=w2799, "输入数据"=w2813) -> ()  [unwired: 1 in, 12 out]
                  }
                }
                n2287 = local write "命令序号"(w2771) -> ()
                n2288 = local write "命令"(w2776) -> ()
                n2289 = local write "清BUFF"(FALSE ("清BUFF")) -> ()
                n2290 = local write "控制1"(TRUE ("控制1")) -> ()
                n2291 = global write "EV05全局变量1.vi" "流控帧 2"(TRUE ("流控帧 2")) -> ()
                n2292 = local write "写?"(FALSE ("写?")) -> ()
                n2293 = local write "消除"(TRUE ("消除")) -> ()
              }
              frame #2 {
                n2294 = flat-sequence {
                  tunnel: [w2819] -> w2818
                  tunnel: w2818 -> [w2826]
                  frame #0 {
                    n2295 = while {
                      tunnel: [w2820] -> w2819
                      i -> [w2824]
                      stop <- w2821 stop-if-true
                      n2296 = local read "继电器超时处理"() -> (w2820:bool)
                      n2297 = Greater Or Equal?(x=w2824, y=20) -> (x >= y?=w2822:bool)
                      n2298 = Wait Until Next ms Multiple(millisecond multiple=u32 100 ("毫秒倍数")) -> ()  [unwired: 1 out]
                      n2299 = Or(x=w2820, y=w2822) -> (x .or. y?=w2821:bool)
                    }
                  }
                  frame #1 {
                    n2300 = case shown="假" w2826 {
                      frame False {
                        n2301 = local read "风机继电器"() -> (w2827:bool)
                        n2302 = Not(x=w2827) -> (.not. x?=w2828:bool)
                        n2303 = local write "风机继电器"(w2828) -> ()
                        n2304 = One Button Dialog(message="继电器处理超时" ("消息"), button name ("OK")="是" ("按钮名称（“确定”）")) -> ()  [unwired: 1 out]
                      }
                      frame True {
                      }
                    }
                  }
                }
              }
            }
          }
          event "加热继电器(从)": Value Change {
            n2305 = event-data() -> ("NewVal"=w2831:bool)  [unwired: 6 out]
            n2306 = stacked-sequence {
              tunnel: w2831 -> [_ w2845 _]
              frame #0 {
                w2835 = FALSE ("继电器超时处理")
                n2307 = local write "正级继电器 7"(w2835) -> ()
                n2308 = local write "继电器超时处理"(w2835) -> ()
                n2309 = global write "EV05全局变量1.vi" "流控帧"(FALSE ("流控帧")) -> ()
                n2310 = local write "主从选择"(enum32{"主板", "从板"}."从板" ("主从选择")) -> ()
              }
              frame #1 {
                n2311 = case shown="真" w2845 {
                  selector: w2845 -> [w2860 w2880]
                  tunnel: [w2859 w2879] -> w2844
                  tunnel: [w2858 w2878] -> w2838
                  tunnel: [w2847 w2867] -> w2839
                  frame True {
                    w2855 = 256.0 ("y")
                    w2847 = u32 1 ("命令序号")
                    w2859 = u8 192 ("命令")
                    n2312 = local read "动作保持时间"() -> (w2856:dbl)
                    n2313 = Quotient & Remainder(x=w2856, y=w2855) -> (x-y*floor(x/y)=w2848:dbl, floor(x/y)=w2852:dbl)
                    n2314 = Quotient & Remainder(x=w2852, y=w2855) -> (x-y*floor(x/y)=w2849:dbl, floor(x/y)=w2853:dbl)
                    n2315 = Quotient & Remainder(x=w2853, y=w2855) -> (x-y*floor(x/y)=w2850:dbl, floor(x/y)=w2854:dbl)
                    n2316 = Quotient & Remainder(x=w2854, y=w2855) -> (x-y*floor(x/y)=w2851:dbl)  [unwired: 1 out]
                    n2317 = Boolean To (0,1)(Boolean=w2860) -> (0, 1=w2857:i16)
                    n2318 = local read "设备索引号"() -> (w2864:u16)
                    n2319 = local read "CAN卡类型"() -> (w2865:u32)
                    n2320 = local read "从板板号"() -> (w2858:u8)
                    n2321 = local read "CAN端口"() -> (w2863:u16)
                    n2322 = Build Array(i16 7 ("元素"), w2857, w2851, w2850, w2849, w2848, 0.0 ("元素")) -> (w2862:dbl[])
                    n2323 = call "多帧发送机制(EV05).vi"("can卡类型"=w2865, "设备索引号"=w2864, "CAN端口"=w2863, "命令"=w2859, "板号"=w2858, "命令序号"=w2847, "输入数据"=w2862) -> ()  [unwired: 1 in, 12 out]
                  }
                  frame False {
                    w2875 = 256.0 ("y")
                    w2867 = u32 1 ("命令序号")
                    w2879 = u8 192 ("命令")
                    n2324 = local read "动作保持时间"() -> (w2876:dbl)
                    n2325 = Quotient & Remainder(x=w2876, y=w2875) -> (x-y*floor(x/y)=w2868:dbl, floor(x/y)=w2872:dbl)
                    n2326 = Quotient & Remainder(x=w2872, y=w2875) -> (x-y*floor(x/y)=w2869:dbl, floor(x/y)=w2873:dbl)
                    n2327 = Quotient & Remainder(x=w2873, y=w2875) -> (x-y*floor(x/y)=w2870:dbl, floor(x/y)=w2874:dbl)
                    n2328 = Quotient & Remainder(x=w2874, y=w2875) -> (x-y*floor(x/y)=w2871:dbl)  [unwired: 1 out]
                    n2329 = Boolean To (0,1)(Boolean=w2880) -> (0, 1=w2877:i16)
                    n2330 = local read "设备索引号"() -> (w2884:u16)
                    n2331 = local read "CAN卡类型"() -> (w2885:u32)
                    n2332 = local read "从板板号"() -> (w2878:u8)
                    n2333 = local read "CAN端口"() -> (w2883:u16)
                    n2334 = Build Array(i16 7 ("元素"), w2877, w2871, w2870, w2869, w2868, 0.0 ("元素")) -> (w2882:dbl[])
                    n2335 = call "多帧发送机制(EV05).vi"("can卡类型"=w2885, "设备索引号"=w2884, "CAN端口"=w2883, "命令"=w2879, "板号"=w2878, "命令序号"=w2867, "输入数据"=w2882) -> ()  [unwired: 1 in, 12 out]
                  }
                }
                n2336 = local write "从板板号"(w2838) -> ()
                n2337 = local write "命令序号"(w2839) -> ()
                n2338 = local write "命令"(w2844) -> ()
                n2339 = local write "清BUFF"(FALSE ("清BUFF")) -> ()
                n2340 = local write "写?"(FALSE ("写?")) -> ()
                n2341 = local write "控制1"(TRUE ("控制1")) -> ()
                n2342 = global write "EV05全局变量1.vi" "流控帧 2"(TRUE ("流控帧 2")) -> ()
                n2343 = local write "消除"(TRUE ("消除")) -> ()
              }
              frame #2 {
                n2344 = flat-sequence {
                  tunnel: [w2887] -> w2886
                  tunnel: w2886 -> [w2894]
                  frame #0 {
                    n2345 = while {
                      tunnel: [w2888] -> w2887
                      i -> [w2892]
                      stop <- w2889 stop-if-true
                      n2346 = local read "继电器超时处理"() -> (w2888:bool)
                      n2347 = Greater Or Equal?(x=w2892, y=20) -> (x >= y?=w2890:bool)
                      n2348 = Wait Until Next ms Multiple(millisecond multiple=u32 100 ("毫秒倍数")) -> ()  [unwired: 1 out]
                      n2349 = Or(x=w2888, y=w2890) -> (x .or. y?=w2889:bool)
                    }
                  }
                  frame #1 {
                    n2350 = case shown="假" w2894 {
                      frame False {
                        n2351 = local read "加热继电器(从)"() -> (w2896:bool)
                        n2352 = Not(x=w2896) -> (.not. x?=w2895:bool)
                        n2353 = local write "加热继电器(从)"(w2895) -> ()
                        n2354 = One Button Dialog(message="继电器处理超时" ("消息"), button name ("OK")="是" ("按钮名称（“确定”）")) -> ()  [unwired: 1 out]
                      }
                      frame True {
                      }
                    }
                  }
                }
              }
            }
          }
          event "风机继电器(从)": Value Change {
            n2355 = event-data() -> ("NewVal"=w2899:bool)  [unwired: 6 out]
            n2356 = stacked-sequence {
              tunnel: w2899 -> [_ w2913 _]
              frame #0 {
                w2903 = FALSE ("继电器超时处理")
                n2357 = local write "继电器超时处理"(w2903) -> ()
                n2358 = local write "正级继电器 8"(w2903) -> ()
                n2359 = global write "EV05全局变量1.vi" "流控帧"(FALSE ("流控帧")) -> ()
                n2360 = local write "主从选择"(enum32{"主板", "从板"}."从板" ("主从选择")) -> ()
              }
              frame #1 {
                n2361 = case shown="假" w2913 {
                  selector: w2913 -> [w2928 w2948]
                  tunnel: [w2927 w2947] -> w2912
                  tunnel: [w2926 w2946] -> w2906
                  tunnel: [w2915 w2935] -> w2907
                  frame False {
                    w2923 = 256.0 ("y")
                    w2915 = u32 1 ("命令序号")
                    w2927 = u8 192 ("命令")
                    n2362 = local read "动作保持时间"() -> (w2924:dbl)
                    n2363 = Quotient & Remainder(x=w2924, y=w2923) -> (x-y*floor(x/y)=w2916:dbl, floor(x/y)=w2920:dbl)
                    n2364 = Quotient & Remainder(x=w2920, y=w2923) -> (x-y*floor(x/y)=w2917:dbl, floor(x/y)=w2921:dbl)
                    n2365 = Quotient & Remainder(x=w2921, y=w2923) -> (x-y*floor(x/y)=w2918:dbl, floor(x/y)=w2922:dbl)
                    n2366 = Quotient & Remainder(x=w2922, y=w2923) -> (x-y*floor(x/y)=w2919:dbl)  [unwired: 1 out]
                    n2367 = local read "设备索引号"() -> (w2932:u16)
                    n2368 = local read "CAN卡类型"() -> (w2933:u32)
                    n2369 = local read "从板板号"() -> (w2926:u8)
                    n2370 = Boolean To (0,1)(Boolean=w2928) -> (0, 1=w2925:i16)
                    n2371 = local read "CAN端口"() -> (w2931:u16)
                    n2372 = Build Array(i16 8 ("元素"), w2925, w2919, w2918, w2917, w2916, 0.0 ("元素")) -> (w2930:dbl[])
                    n2373 = call "多帧发送机制(EV05).vi"("can卡类型"=w2933, "设备索引号"=w2932, "CAN端口"=w2931, "命令"=w2927, "板号"=w2926, "命令序号"=w2915, "输入数据"=w2930) -> ()  [unwired: 1 in, 12 out]
                  }
                  frame True {
                    w2943 = 256.0 ("y")
                    w2935 = u32 1 ("命令序号")
                    w2947 = u8 192 ("命令")
                    n2374 = local read "动作保持时间"() -> (w2944:dbl)
                    n2375 = Quotient & Remainder(x=w2944, y=w2943) -> (x-y*floor(x/y)=w2936:dbl, floor(x/y)=w2940:dbl)
                    n2376 = Quotient & Remainder(x=w2940, y=w2943) -> (x-y*floor(x/y)=w2937:dbl, floor(x/y)=w2941:dbl)
                    n2377 = Quotient & Remainder(x=w2941, y=w2943) -> (x-y*floor(x/y)=w2938:dbl, floor(x/y)=w2942:dbl)
                    n2378 = Quotient & Remainder(x=w2942, y=w2943) -> (x-y*floor(x/y)=w2939:dbl)  [unwired: 1 out]
                    n2379 = local read "设备索引号"() -> (w2952:u16)
                    n2380 = local read "CAN卡类型"() -> (w2953:u32)
                    n2381 = local read "从板板号"() -> (w2946:u8)
                    n2382 = Boolean To (0,1)(Boolean=w2948) -> (0, 1=w2945:i16)
                    n2383 = local read "CAN端口"() -> (w2951:u16)
                    n2384 = Build Array(i16 8 ("元素"), w2945, w2939, w2938, w2937, w2936, 0.0 ("元素")) -> (w2950:dbl[])
                    n2385 = call "多帧发送机制(EV05).vi"("can卡类型"=w2953, "设备索引号"=w2952, "CAN端口"=w2951, "命令"=w2947, "板号"=w2946, "命令序号"=w2935, "输入数据"=w2950) -> ()  [unwired: 1 in, 12 out]
                  }
                }
                n2386 = local write "从板板号"(w2906) -> ()
                n2387 = local write "清BUFF"(FALSE ("清BUFF")) -> ()
                n2388 = local write "命令序号"(w2907) -> ()
                n2389 = local write "命令"(w2912) -> ()
                n2390 = local write "控制1"(TRUE ("控制1")) -> ()
                n2391 = local write "写?"(FALSE ("写?")) -> ()
                n2392 = local write "消除"(TRUE ("消除")) -> ()
                n2393 = global write "EV05全局变量1.vi" "流控帧 2"(TRUE ("流控帧 2")) -> ()
              }
              frame #2 {
                n2394 = flat-sequence {
                  tunnel: [w2955] -> w2954
                  tunnel: w2954 -> [w2962]
                  frame #0 {
                    n2395 = while {
                      tunnel: [w2956] -> w2955
                      i -> [w2960]
                      stop <- w2957 stop-if-true
                      n2396 = local read "继电器超时处理"() -> (w2956:bool)
                      n2397 = Greater Or Equal?(x=w2960, y=20) -> (x >= y?=w2958:bool)
                      n2398 = Wait Until Next ms Multiple(millisecond multiple=u32 100 ("毫秒倍数")) -> ()  [unwired: 1 out]
                      n2399 = Or(x=w2956, y=w2958) -> (x .or. y?=w2957:bool)
                    }
                  }
                  frame #1 {
                    n2400 = case shown="假" w2962 {
                      frame False {
                        n2401 = local read "风机继电器(从)"() -> (w2964:bool)
                        n2402 = Not(x=w2964) -> (.not. x?=w2963:bool)
                        n2403 = local write "风机继电器(从)"(w2963) -> ()
                        n2404 = One Button Dialog(message="继电器处理超时" ("消息"), button name ("OK")="是" ("按钮名称（“确定”）")) -> ()  [unwired: 1 out]
                      }
                      frame True {
                      }
                    }
                  }
                }
              }
            }
          }
          event "DO1": Value Change {
            n2405 = event-data() -> ("NewVal"=w2967:bool)  [unwired: 6 out]
            n2406 = stacked-sequence {
              tunnel: w2967 -> [_ w2980 _]
              frame #0 {
                w2970 = FALSE ("清BUFF")
                n2407 = local write "继电器超时处理"(FALSE ("继电器超时处理")) -> ()
                n2408 = local write "清BUFF"(w2970) -> ()
